vi "mfFreqDev.vi"(8 "error in (no error)":errorcluster caption="错误输入（无错误）", 10 "pichData":cdb[](array[numeric]), 11 "Path":path) -> (0 "error out":errorcluster caption="错误输出", 3 "devVal":dbl)   [LabVIEW 2015]
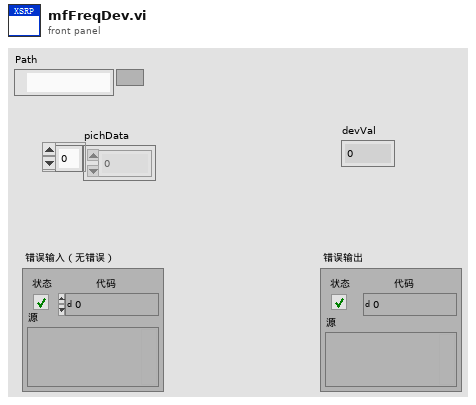
[diagram p1: front panel]
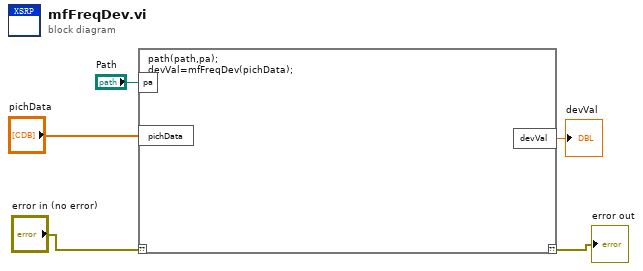
[diagram p0: block diagram]
diagram:
  n1 = script code="path(path,pa);\ndevVal=mfFreqDev(pichData);"("??"="error in (no error)", "pa"="Path", "pichData"="pichData") -> ("??"=→"error out":errorcluster, "devVal"=→"devVal":dbl)
